vi "test_Copy LogFile from Target.vi"(8 "error in (no error)":errorcluster, 11 "TestCase in":refnum<class "Telemetry System Tests.lvclass">=refnum) -> (0 "error out":errorcluster, 3 "TestCase out":refnum<class "Telemetry System Tests.lvclass">)   [LabVIEW 2026, in "Telemetry System Tests.lvclass"]
uses:
  Telemetry System Tests.lvclass
  Telemetry System Tests.lvclass/Telemetry System Tests.ctl
  Telemetry Test Utilities/Telemetry Test Utilities.lvlib
  b15e678b-00b4-460c-84a3-511904b6b81c.vi
  bea3641c-2db6-4d0f-ba30-d41bc63e0e70.vi
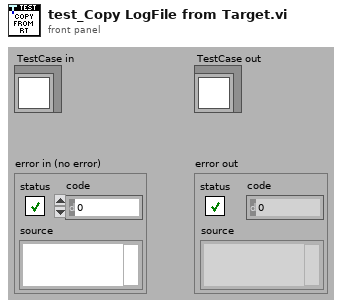
[diagram p1: front panel]
types:
  T1 = typedef "VeriStandTestUtilities.lvlib/TargetInformation.ctl" = cluster{"Name":string, "IP Address":string, "Operating System":string, "Target Rate":dbl, "Chassis List":T2[], "Custom Device List":string[]}
  T2 = typedef "VeriStandTestUtilities.lvlib/ChassisInformation.ctl" = cluster{"Name":string, "Devices":string[]}
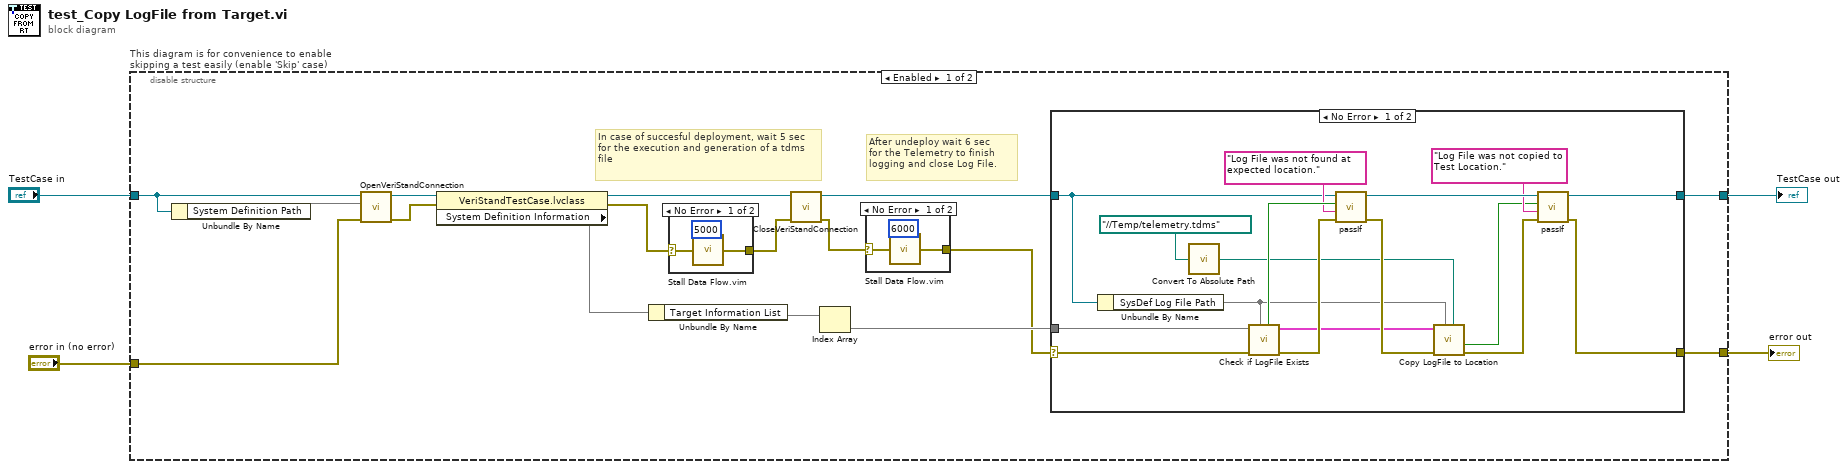
[diagram p0: block diagram]
diagram:
  n1 = disable-structure "This diagram is for convenience to enable skipping a test easily (enable 'Skip' case)" shown="Enabled" {
    disable-tunnel: "TestCase in" -> [w15 w51]
    disable-tunnel: [w19 w49] -> w1
    disable-tunnel: [w20 w50] -> w3
    disable-tunnel: "error in (no error)" -> [w18 w48]
    frame Enabled {
      # "After undeploy wait 6 sec\nfor the Telemetry to finish logging and close Log File."
      # "In case of succesful deployment, wait 5 sec for the execution and generation of a tdms file"
      n2 = Unbundle By Name(w15) -> ("System Definition Path"=w14)
      n3 = call-dynamic "OpenVeriStandConnection.vi"("error in (no error)"=w18, "System Definition File"=w14, "VeriStand Test Case in"=w15) -> ("error out"=w13:errorcluster, "VeriStand Test Case out"=w12:refnum<class "VeriStandTestCase.lvclass">)  [unwired: 6 in, 1 out]
      n4 = property class="VeriStandTestCase.lvclass"(reference=w12, error in=w13) -> (reference out=w11:refnum<class "VeriStandTestCase.lvclass">, error out=w10:errorcluster, "System Definition Information"=w8)
      n5 = Unbundle By Name(w8) -> ("Target Information List"=w9)
      n6 = case shown="No Error" w10 {
        selector: w10 -> [w27 w28]
        tunnel: [w25 w28] -> w16
        frame No Error {
          n7 = call "Stall Data Flow.vim"("value in"=w27, "milliseconds to wait"=u32 5000) -> ("value out"=w25:errorcluster)  [unwired: 1 out]
        }
        frame Error {
        }
      }
      n8 = call-dynamic "CloseVeriStandConnection.vi"("error in (no error)"=w16, "VeriStand Test Case in"=w11) -> ("error out"=w6:errorcluster, "VeriStand Test Case out"=w17:refnum<class "VeriStandTestCase.lvclass">)  [unwired: 8 in]
      n9 = Index Array(array=w9) -> (element=w7)  [unwired: 1 in]
      n10 = case shown="No Error" w6 {
        selector: w6 -> [w23 w24]
        tunnel: [w21 w24] -> w5
        frame No Error {
          n11 = call "Stall Data Flow.vim"("value in"=w23, "milliseconds to wait"=u32 6000) -> ("value out"=w21:errorcluster)  [unwired: 1 out]
        }
        frame Error {
        }
      }
      n12 = case shown="No Error" w5 {
        selector: w5 -> [w35 w47]
        tunnel: [w38 w47] -> w20
        tunnel: [w37 w46] -> w19
        tunnel: w17 -> [w32 w46]
        tunnel: w7 -> [w36 _]
        frame No Error {
          n13 = Unbundle By Name(w32) -> ("SysDef Log File Path"=w31)
          n14 = call "Convert To Absolute Path.vi"("System Definition File Path"=path "../../Temp/telemetry.tdms" ("relative base path")) -> ("Absolute path"=w41:path)
          n15 = call "Check if LogFile Exists.vi"("Log File Path"=w31, "error in (no error)"=w35, "Target Information"=w36) -> ("error out"=w45:errorcluster, "Target Information out"=w30:T1, "LogFile Exists?"=w44:bool)  [unwired: 6 in]
          n16 = call-dynamic "passIf.vi"("error in (no error)"=w45, "message (\"\")"="Log File was not found at expected location." ("message (\"\")"), "pass"=w44, "TestCase in"=w32) -> ("error out"=w43:errorcluster, "TestCase out"=w40:refnum<class "Telemetry System Tests.lvclass">)  [unwired: 6 in]
          n17 = call "Copy LogFile to Location.vi"("Local Save Path in"=w41, "Log File Path in"=w31, "error in"=w43, "Target Information in"=w30) -> ("error out"=w39:errorcluster, "File Succesfuly copied"=w29:bool)  [unwired: 4 in, 2 out]
          n18 = call-dynamic "passIf.vi"("error in (no error)"=w39, "message (\"\")"="Log File was not copied to Test Location." ("message (\"\")"), "pass"=w29, "TestCase in"=w40) -> ("error out"=w38:errorcluster, "TestCase out"=w37:refnum<class "Telemetry System Tests.lvclass">)  [unwired: 6 in]
        }
        frame Error {
        }
      }
    }
    frame Disabled {
      # "skip test result while test is under development"
      n19 = call <vilib>:"skip.vi"("error in (no error)"=w48, "TestCase in"=w51) -> ("error out"=w50:errorcluster, "TestCase out"=w49:refnum<class "Telemetry System Tests.lvclass">)  [unwired: 8 in]
    }
  }
  "error out" <- w3
  "TestCase out" <- w1
